vi "Find Msgs.vi"(11 "Base Actor in":refnum<class "Base Actor.lvclass">) -> (2 "Msgs":T1)   [LabVIEW 2020, in "jettl.lvlib" / "Base jettl Actor.lvlib" / "Base Actor.lvlib" / "Base Actor.lvclass"]
uses:
  Base Actor.lvclass
  Base Actor.lvclass/Base Actor.ctl
  jettl.lvlib
  Msg/Msg.lvclass
  Msg Set.ctl
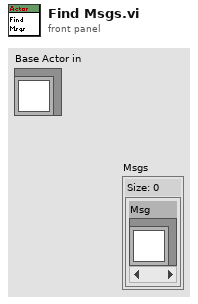
[diagram p1: front panel]
types:
  T1 = typedef "jettl.lvlib/Msg Set.ctl" = set{refnum<class "Msg.lvclass">}
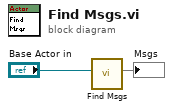
[diagram p0: block diagram]
diagram:
  n1 = call "Find Msgs.vi"("X Actor.lvclass"="Base Actor in") -> ("Msgs"=→"Msgs":T1)  [unwired: 10 in]
